vi "Update FL Channels.vi"(8 "error in (no error)":errorcluster, 11 "Performanced XNET CAN Signal Logger in":refnum<class "Performanced XNET CAN Signal Logger.lvclass">) -> (0 "error out":errorcluster, 3 "Performanced XNET CAN Signal Logger out":refnum<class "Performanced XNET CAN Signal Logger.lvclass">)   [LabVIEW 2021, in "Performanced XNET CAN Signal Logger.lvlib" / "Performanced XNET CAN Signal Logger.lvclass"]
uses:
  Performanced XNET CAN Signal Logger.lvclass
  C:/Program Files/National Instruments/LabVIEW 2021/vi.lib/FlexLogger/SDK/PluginSDK.lvlibp/PEFClasses/SDK/Plugin/Plugin.lvclass
  C:/Program Files/National Instruments/LabVIEW 2021/vi.lib/FlexLogger/SDK/PluginSDK.lvlibp/PEFClasses/SDK/Processing Element/Processing Element.lvclass
  <vilib>/FlexLogger/SDK/PluginSDK.lvlibp/PEFClasses/SDK/Processing Element/Read System Interface.vi
  <vilib>/FlexLogger/SDK/PluginSDK.lvlibp/PEFClasses/SDK/Plugin/Read Channels.vi
  <vilib>/FlexLogger/SDK/PluginSDK.lvlibp/PEFClasses/SDK/Channel/ParameterAccess/Read Enum.vi
  <vilib>/FlexLogger/SDK/PluginSDK.lvlibp/PEFClasses/SDK/Channel/Write Unit.vi
  <vilib>/FlexLogger/SDK/PluginSDK.lvlibp/PEFClasses/SDK/Addon Interface/Addon Interface.lvclass
  <vilib>/FlexLogger/SDK/PluginSDK.lvlibp/PEFClasses/SDK/System Interface/System Interface.lvclass
  <vilib>/FlexLogger/SDK/PluginSDK.lvlibp/PEFClasses/SDK/Channel/Channel.lvclass
  Performanced XNET CAN Signal Logger.lvclass/Performanced XNET CAN Signal Logger.ctl
  <vilib>/FlexLogger/SDK/PluginSDK.lvlibp
  <vilib>/FlexLogger/SDK/PluginSDK.lvlibp/PEFClasses/SDK/Channel/ParameterAccess/Write Enum.vi
  <vilib>/FlexLogger/SDK/PluginSDK.lvlibp/PEFClasses/SDK/Plugin/Plugin.lvclass
  <vilib>/FlexLogger/SDK/PluginSDK.lvlibp/PEFClasses/SDK/Producer Channel/Create Producer Channel.vi
  <vilib>/FlexLogger/SDK/PluginSDK.lvlibp/PEFClasses/SDK/Producer Channel/Producer Channel.lvclass
  C:/Program Files/National Instruments/LabVIEW 2021/vi.lib/FlexLogger/SDK/PluginSDK.lvlibp/PEFClasses/SDK/Channel/Channel.lvclass
  C:/Program Files/National Instruments/LabVIEW 2021/vi.lib/FlexLogger/SDK/PluginSDK.lvlibp/PEFClasses/SDK/Producer Channel/Producer Channel.lvclass
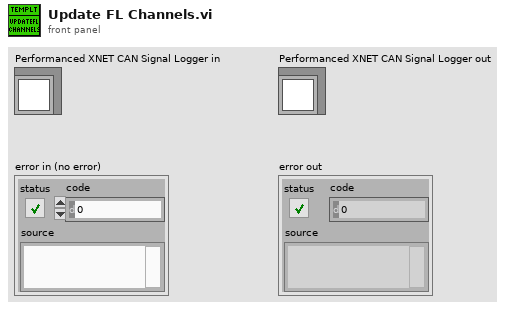
[diagram p1: front panel]
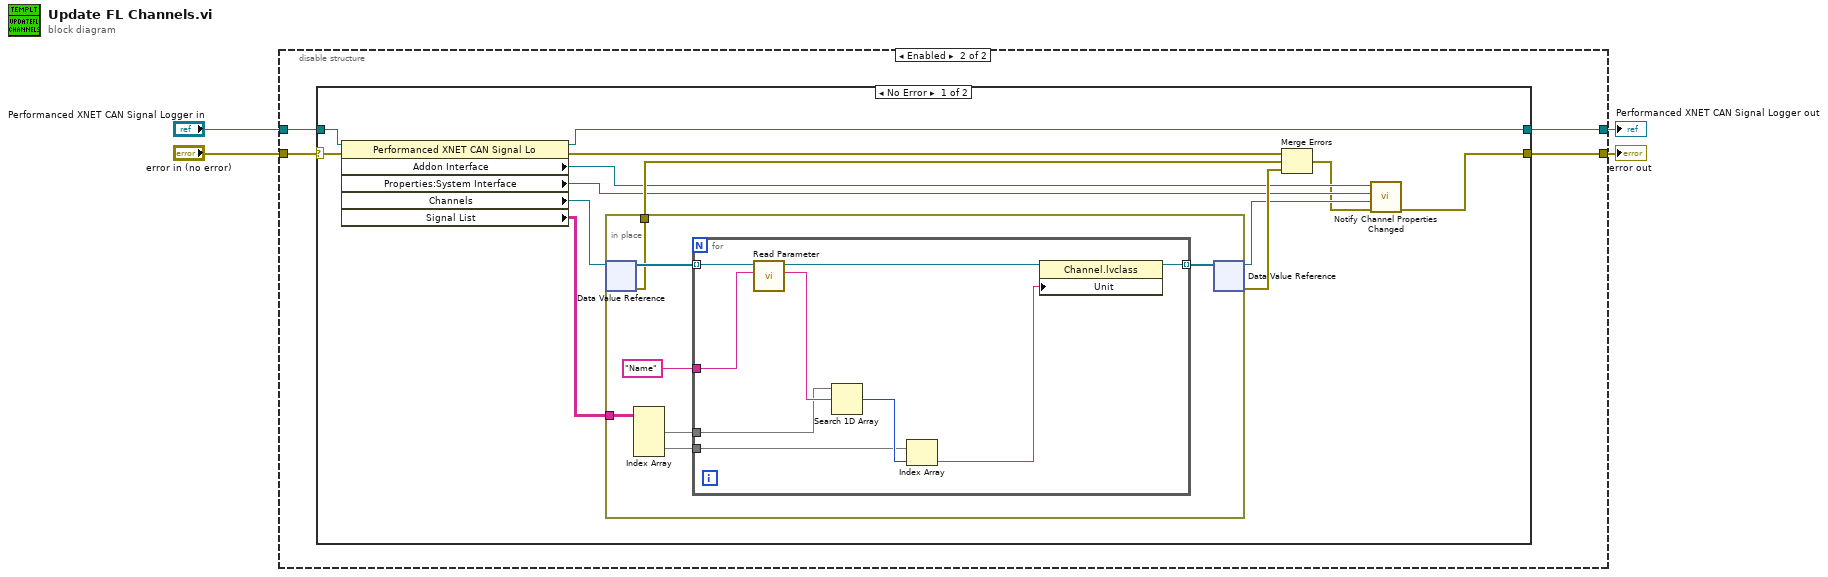
[diagram p0: block diagram]
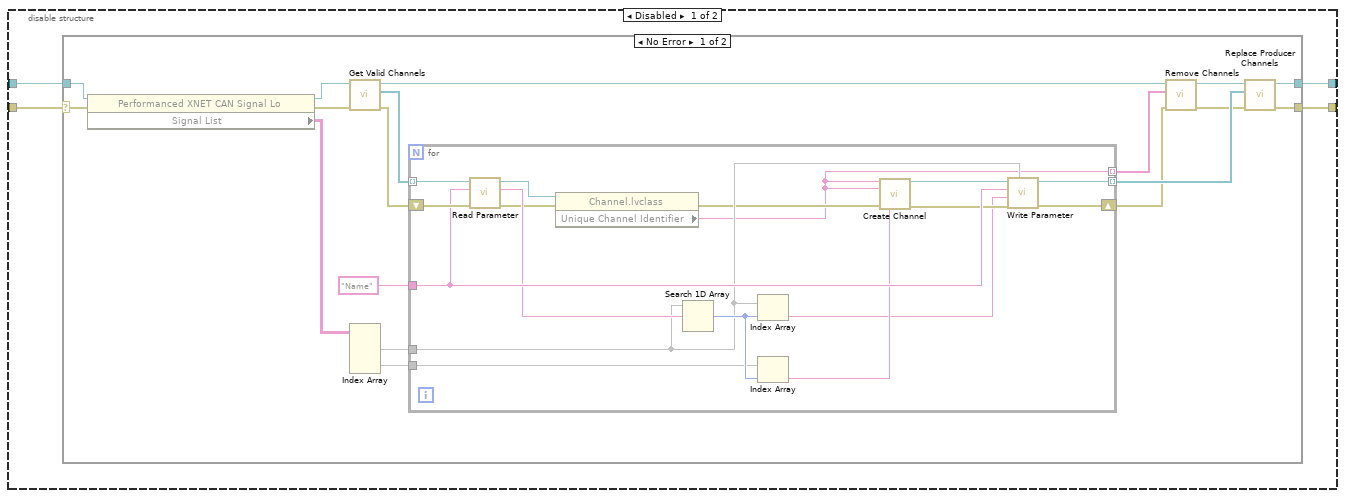
[diagram p2: hidden frame]
diagram:
  n1 = disable-structure shown="Enabled" {
    disable-tunnel: "Performanced XNET CAN Signal Logger in" -> [w8 w49]
    disable-tunnel: "error in (no error)" -> [w7 w48]
    disable-tunnel: [w6 w47] -> w2
    disable-tunnel: [w5 w46] -> w1
    frame Disabled {
      n2 = case shown="No Error" w7 {
        selector: w7 -> [w25 w44]
        tunnel: [w23 w45] -> w6
        tunnel: [w22 w44] -> w5
        tunnel: w8 -> [w24 w45]
        frame No Error {
          n3 = property class="Performanced XNET CAN Signal Lo"(reference=w24, error in=w25) -> (reference out=w26:refnum<class "Performanced XNET CAN Signal Logger.lvclass">, error out=w14:errorcluster, "Signal List"=w18:string[][])
          n4 = call <vilib>:"Get Valid Channels.vi"("error in (no error)"=w14, "Plugin in"=w26) -> ("error out"=w13:errorcluster, "Channels"=w15:refnum<class "Channel.lvclass">[], "Plugin out"=w16:refnum<class "Performanced XNET CAN Signal Logger.lvclass">)  [unwired: 7 in]
          n5 = Index Array(array=w18) -> (element #1=w19:string[], element #2=w20:string[])  [unwired: 4 in]
          n6 = for {
            tunnel: w15 -> [w43] mode=indexing
            tunnel: w19 -> [w32]
            tunnel: "Name" ("Name") -> [w39]
            tunnel: w20 -> [w37]
            shift-right: [w40] -> w11
            shift-left: w13 -> [w41]
            tunnel: [w29] -> w17 mode=indexing
            tunnel: [w27] -> w9 mode=indexing
            n7 = call-poly <vilib>:"Read Parameter.vi"("error in (no error)"=w41, "Name"=w39, "Channel in"=w43) -> ("error out"=w35:errorcluster, "Value"=w38:string, "Channel out"=w30:refnum<class "Channel.lvclass">)  [unwired: 4 in, 2 out]
            n8 = property class="Channel.lvclass"(reference=w30, error in=w35) -> (error out=w31:errorcluster, "Unique Channel Identifier"=w27:string)  [unwired: 1 out]
            n9 = Search 1D Array(1D array=w32, element=w38) -> (index of element=w42:i32)  [unwired: 1 in]
            n10 = Index Array(array=w32, index=w42) -> (element=w28:string)
            n11 = Index Array(array=w37, index=w42) -> (element=w34:string)
            n12 = call-poly <vilib>:"Create Channel.vi"("Unique Channel Identifier"=w27, "Default Channel Name"=w27, "error in (no error)"=w31, "Unit"=w34) -> ("Producer Channel"=w36:refnum<class "Producer Channel.lvclass">, "error out"=w33:errorcluster)  [unwired: 10 in]
            n13 = call-poly <vilib>:"Write Parameter.vi"("Possible Values"=w32, "error in (no error)"=w33, "Current Value"=w28, "Name"=w39, "Channel in"=w36) -> ("error out"=w40:errorcluster, "Channel out"=w29:refnum<class "Producer Channel.lvclass">)  [unwired: 5 in]
          }
          n14 = call-dynamic "Remove Channels.vi"("error in (no error)"=w11, "Unique Channel Identifiers to Delete"=w9, "Plugin in"=w16) -> ("error out"=w10:errorcluster, "Plugin out"=w12:refnum<class "Performanced XNET CAN Signal Logger.lvclass">)  [unwired: 7 in]
          n15 = call <vilib>:"Replace Producer Channels.vi"("error in (no error)"=w10, "Producer Channels"=w17, "Plugin"=w12) -> ("error out"=w22:errorcluster, "Plugin"=w23:refnum<class "Performanced XNET CAN Signal Logger.lvclass">)  [unwired: 7 in]
        }
        frame Error {
        }
      }
    }
    frame Enabled {
      n16 = case shown="No Error" w48 {
        selector: w48 -> [w62 w79]
        tunnel: [w55 w80] -> w47
        tunnel: [w50 w79] -> w46
        tunnel: w49 -> [w61 w80]
        frame No Error {
          n17 = property class="Performanced XNET CAN Signal Lo"(reference=w61, error in=w62) -> (reference out=w55:refnum<class "Performanced XNET CAN Signal Logger.lvclass">, error out=w58:errorcluster, "Addon Interface"=w53:refnum<class "Addon Interface.lvclass">, "Properties:System Interface"=w54:refnum<class "System Interface.lvclass">, "Channels"=w59:refnum<data-value>, "Signal List"=w60:string[][])
          n18 = in-place {
            in-place-border: w60 -> [w66]
            in-place-border: [w63] -> w57
            n19 = in-place-dvr #1(w59) -> (w65:refnum<class "Channel.lvclass">[], w63:errorcluster)
            n20 = Index Array(array=w66) -> (element #1=w67:string[], element #2=w68:string[])  [unwired: 4 in]
            n21 = for {
              tunnel: w67 -> [w74]
              tunnel: "Name" ("Name") -> [w77]
              tunnel: w68 -> [w75]
              tunnel: [w71] -> w64 mode=indexing
              tunnel: w65 -> [w72] mode=indexing
              n22 = call-poly <vilib>:"Read Parameter.vi"("Name"=w77, "Channel in"=w72) -> ("Value"=w76:string, "Channel out"=w73:refnum<class "Channel.lvclass">)  [unwired: 5 in, 3 out]
              n23 = Search 1D Array(1D array=w74, element=w76) -> (index of element=w78:i32)  [unwired: 1 in]
              n24 = Index Array(array=w75, index=w78) -> (element=w70:string)
              n25 = property class="Channel.lvclass"(reference=w73, "Unit"=w70) -> (reference out=w71:refnum<class "Channel.lvclass">)  [unwired: 1 in, 1 out]
            }
            n26 = in-place-dvr #1(w64) -> (w52:refnum<data-value>, w56:errorcluster)
          }
          n27 = Merge Errors(w58, w57, w56) -> (w51:errorcluster)
          n28 = call-dynamic "Notify Channel Properties Changed.vi"("error in (no error)"=w51, "Channels DVR"=w52, "System Interface in"=w54, "Addon Interface in"=w53) -> ("error out"=w50:errorcluster)  [unwired: 5 in, 2 out]
        }
        frame Error {
        }
      }
    }
  }
  "Performanced XNET CAN Signal Logger out" <- w2
  "error out" <- w1
